vi "run.vi"(8 "error in (no error)":errorcluster, 11 "GenericMicroscope in":refnum<class "GenericInstrument.lvclass">) -> (0 "error out":errorcluster, 3 "GenericMicroscope out":refnum<class "GenericInstrument.lvclass">)   [LabVIEW 2010, in "GenericInstrument.lvclass"]
uses:
  GenericInstrument.lvclass
  main/labview_source/type_definitions/enumerations/main_trigger_enum.ctl
panel:
  # "Functionality not available..."
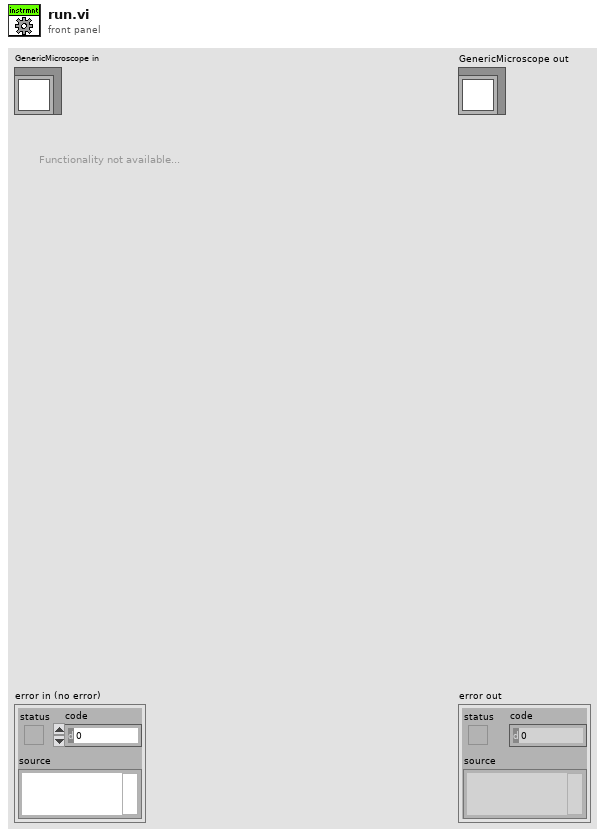
[diagram p1: front panel]
types:
  T1 = typedef "main_trigger_enum.ctl" = enum16{"NULL", "initialise", "terminate", "start", "stop", "change objective", "change experimentController", "change imagingMode", "save notebook", "started saving", "finished saving", "expCtr ready", "expCtr missing", "imgMd ready", "imgMd missing", "scanHd ready", "scanHd missing", "DAQ ready", "DAQ missing", "imgAsm ready", "imgAsm missing", "dataColl ready", "dataColl missing", "display ready", "display missing", "analysr ready", "analysr missing", "instrmnt ready", "instrmnt missing", "stimltr ready", "stimltr missing", "stage ready", "stage missing"}
  T2 = typedef "GenericToplevelComponent.lvclass/common_trigger_enum.ctl" = enum16{"NULL", "initialise", "terminate", "fetch command", "fetch data", "attach observer", "register as observer", "detach observer", "acknowledge", "start", "stop", "sweep started", "sweep finished", "experiment started", "experiment stopped"}
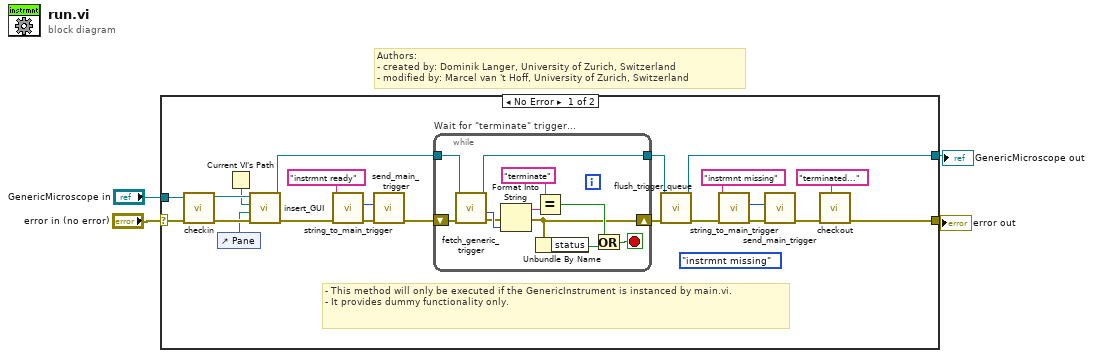
[diagram p0: block diagram]
diagram:
  # "Authors: \n- created by: Dominik Langer, University of Zurich, Switzerland\n- modified by: Marcel van 't Hoff, University of Zurich, Switzerland"
  n1 = case shown="No Error" "error in (no error)" {
    selector: "error in (no error)" -> [w26 w39]
    tunnel: [w25 w39] -> w3
    tunnel: [w14 w38] -> w1
    tunnel: "GenericMicroscope in" -> [w24 w38]
    frame No Error {
      (unwired) main_trigger_enum."instrmnt missing" ("trigger")
      # "- This method will only be executed if the GenericInstrument is instanced by main.vi.\n- It provides dummy functionality only."
      n2 = call-dynamic "checkin.vi"("error in (no error)"=w26, "GenericMicroscope in"=w24) -> ("error out"=w21:errorcluster, "GenericMicroscope out"=w20:refnum<class "GenericInstrument.lvclass">)  [unwired: 8 in]
      n3 = control-ref of="Pane"() -> (w18:refnum<vi>)
      n4 = Current VI's Path() -> (path=w19:path)
      n5 = call-dynamic "insert_GUI.vi"("error in (no error)"=w21, "Pane"=w18, "VI path"=w19, "GenericComponent in"=w20) -> ("error out"=w12:errorcluster, "GenericComponent out"=w16:refnum<class "GenericInstrument.lvclass">)  [unwired: 6 in]
      n6 = call "string_to_main_trigger.vi"("error in (no error)"=w12, "trigger string"="instrmnt ready") -> ("error out"=w11:errorcluster, "main trigger"=w10:T1)  [unwired: 8 in]
      n7 = call "send_main_trigger.vi"("error in (no error)"=w11, "trigger"=w10) -> ("error out"=w22:errorcluster)  [unwired: 9 in]
      n8 = while "Wait for \"terminate\" trigger..." {
        shift-right: [w29] -> w17
        shift-left: w22 -> [w37]
        tunnel: w16 -> [w36]
        tunnel: [w32] -> w15
        stop <- w33 stop-if-true
        n9 = call-dynamic "fetch_generic_trigger.vi"("error in (no error)"=w37, "GenericToplevelComponent in"=w36) -> ("error out"=w30:errorcluster, "common trigger"=w31:T2, "GenericToplevelComponent out"=w32:refnum<class "GenericInstrument.lvclass">)  [unwired: 3 in, 4 out]
        n10 = Format Into String(error in=w30, w31) -> (resulting string=w28:string, error out=w29:errorcluster)  [unwired: 2 in]
        n11 = Equal?(x="terminate", y=w28) -> (x = y?=w34:bool)
        n12 = Unbundle By Name(w29) -> ("status"=w35:bool)
        n13 = Or(x=w34, y=w35) -> (x .or. y?=w33:bool)
      }
      n14 = call-dynamic "flush_trigger_queue.vi"("error in (no error)"=w17, "GenericToplevelComponent in"=w15) -> ("error out"=w8:errorcluster, "GenericToplevelComponent out"=w14:refnum<class "GenericInstrument.lvclass">)  [unwired: 8 in]
      n15 = call "string_to_main_trigger.vi"("error in (no error)"=w8, "trigger string"="instrmnt missing") -> ("error out"=w7:errorcluster, "main trigger"=w5:T1)  [unwired: 8 in]
      n16 = call "send_main_trigger.vi"("error in (no error)"=w7, "trigger"=w5) -> ("error out"=w23:errorcluster)  [unwired: 9 in]
      n17 = call "checkout.vi"("locked by?"="terminated...", "error in (no error)"=w23) -> ("error out"=w25:errorcluster)  [unwired: 8 in, 1 out]
    }
    frame Error {
    }
  }
  "error out" <- w3
  "GenericMicroscope out" <- w1
